vi "Flash LED.vi"(4 "에러 입력(에러 없음)":errorcluster, 7 "Bool 참조번호":refnum<vi>) -> (0 "에러 출력":errorcluster)   [LabVIEW 2018]
doc: "This VI is a subVI for an exercise in the LabVIEW Advanced course."
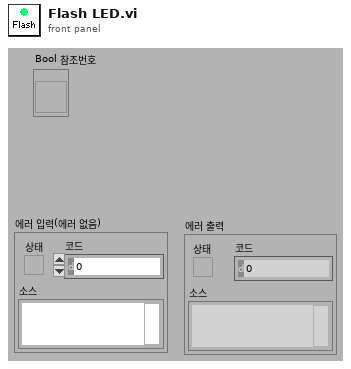
[diagram p1: front panel]
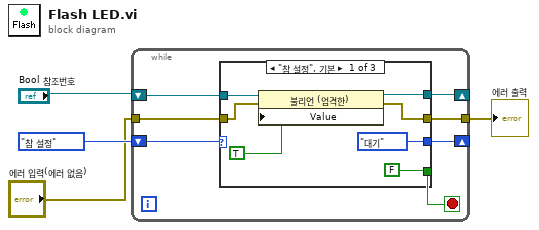
[diagram p0: block diagram]
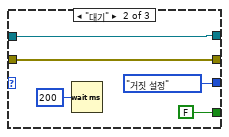
[diagram p2: hidden frame]
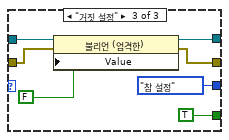
[diagram p3: hidden frame]
diagram:
  n1 = while {
    shift-right: [w9] -> _
    shift-left: "Bool 참조번호" -> [w10]
    shift-right: [w8] -> _
    shift-left: enum16{"참 설정", "대기", "거짓 설정"}."참 설정" -> [w11]
    tunnel: "에러 입력(에러 없음)" -> [w6]
    tunnel: [w5] -> w1
    stop <- w7 stop-if-true
    n2 = case shown="\"참 설정\", 기본" w11 {
      tunnel: w10 -> [w18 w22 w30]
      tunnel: [w16 w22 w29] -> w9
      tunnel: [enum16{"참 설정", "대기", "거짓 설정"}."대기" enum16{"참 설정", "대기", "거짓 설정"}."거짓 설정" enum16{"참 설정", "대기", "거짓 설정"}."참 설정"] -> w8
      tunnel: [FALSE ("값") FALSE ("값") TRUE ("값")] -> w7
      tunnel: w6 -> [w13 w21 w27]
      tunnel: [w12 w21 w28] -> w5
      frame "참 설정", Default {
        n3 = property class="불리언 (엄격한)"(reference=w18, error in=w13, "Value"=TRUE ("값")) -> (reference out=w16:refnum<vi>, error out=w12:errorcluster)
      }
      frame "대기" {
        n4 = Wait (ms)(milliseconds to wait=u32 200 ("기다릴 ms")) -> ()  [unwired: 1 out]
      }
      frame "거짓 설정" {
        n5 = property class="불리언 (엄격한)"(reference=w30, error in=w27, "Value"=FALSE ("값")) -> (reference out=w29:refnum<vi>, error out=w28:errorcluster)
      }
    }
  }
  "에러 출력" <- w1
